vi "Lab4.vi"() -> ()   [LabVIEW 2021]
panel:
  in  "Frequency":dbl(slide) scale=0.0..5.0
  in  "Amplitude":dbl(slide) scale=0.0..10.0
  out "Waveform Chart":dbl(graph)
  in  "stop":bool
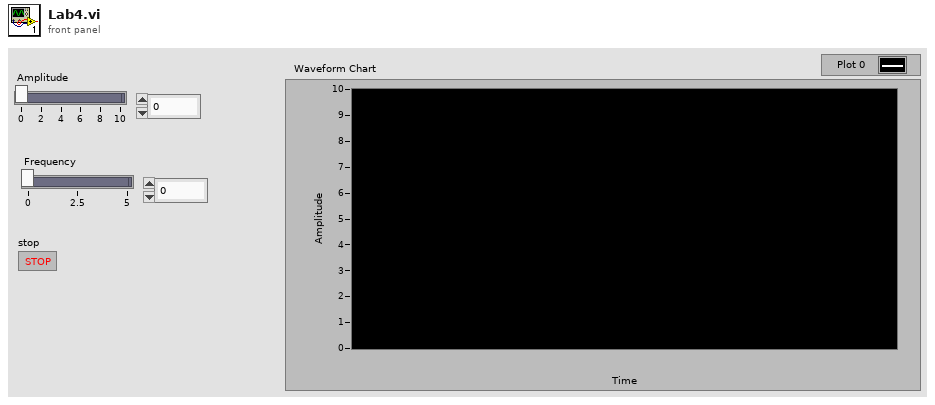
[diagram p1: front panel]
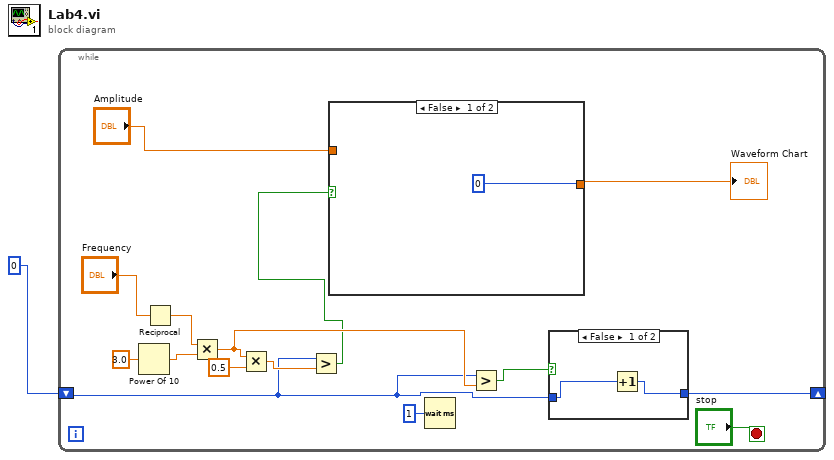
[diagram p0: block diagram]
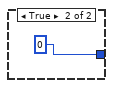
[diagram p2: hidden frame]
diagram:
  n1 = while {
    shift-right: [w11] -> _
    shift-left: 0 -> [w8]
    stop <- "stop" stop-if-true
    n2 = Power Of 10(x=3.0) -> (10^x=w7:dbl)
    n3 = Reciprocal(x="Frequency") -> (1/x=w16:dbl)
    n4 = Multiply(x=w16, y=w7) -> (x*y=w12:dbl)
    n5 = Multiply(x=w12, y=0.5) -> (x*y=w14:dbl)
    n6 = Greater?(x=w8, y=w14) -> (0:w9:bool)
    n7 = case shown="False" w9 {
      tunnel: [0 w21] -> w5
      tunnel: "Amplitude" -> [_ w21]
      frame False {
      }
      frame True {
      }
    }
    "Waveform Chart" <- w5
    n8 = Wait (ms)(milliseconds to wait=u32 1) -> ()  [unwired: 1 out]
    n9 = Greater?(x=w8, y=w12) -> (0:w13:bool)
    n10 = case shown="False" w13 {
      tunnel: [w18 0] -> w11
      tunnel: w8 -> [w17 _]
      frame False {
        n11 = Increment(x=w17) -> (x+1=w18:i32)
      }
      frame True {
      }
    }
  }
